vi "times_called.vi"(2 "reset?":bool) -> (7 "times called":i32)   [LabVIEW 2015]
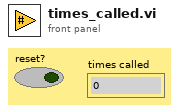
[diagram p1: front panel]
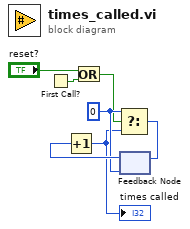
[diagram p0: block diagram]
diagram:
  w5 = 0
  n1 = First Call?() -> (First Call?: T/F=w1:bool)
  n2 = Or(x="reset?", y=w1) -> (x .or. y?=w2:bool)
  n3 = feedback #1(w5) -> (w7:i32)
  n4 = Increment(x=w7) -> (x+1=w4:i32)
  "times called" <- w4
  n5 = Select(t=w5, s=w2, f=w4) -> (s? t:f=w6:i32)
  n6 = feedback-in #1(w6) -> ()
